vi "Increment Subscribers.vi"(8 "error in (no error)":errorcluster, 11 "CIFChannels in":refnum<class "CIFChannels.lvclass">) -> (0 "error out":errorcluster, 3 "CIFChannels out":refnum<class "CIFChannels.lvclass">)   [LabVIEW 2021, in "CIFChannels.lvclass"]
uses:
  CIFChannels.lvclass
  CIFChannels.lvclass/CIFChannels.ctl
  Typedef/Channel State.ctl
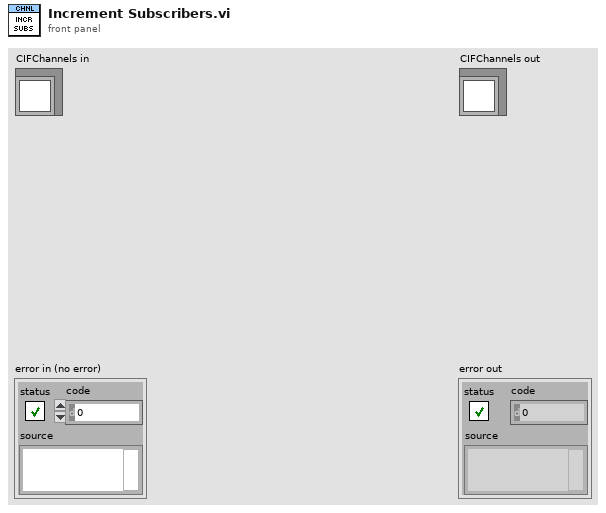
[diagram p1: front panel]
types:
  T1 = typedef "CIFChannels.lvclass/Channel State.ctl" = enum16{"Creating", "Disconnected", "Connecting", "Connected", "Destroyed"}
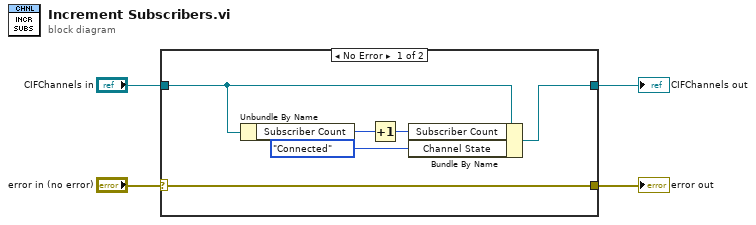
[diagram p0: block diagram]
diagram:
  n1 = case shown="No Error" "error in (no error)" {
    selector: "error in (no error)" -> [w10 w12]
    tunnel: [w10 w12] -> w3
    tunnel: [w5 w11] -> w1
    tunnel: "CIFChannels in" -> [w8 w11]
    frame No Error {
      n2 = Unbundle By Name(w8) -> ("Subscriber Count"=w9:u32)
      n3 = Increment(x=w9) -> (x+1=w7:u32)
      n4 = Bundle By Name(cluster=w8, "Subscriber Count"=w7, "Channel State"=Channel_State."Connected") -> (w5:refnum<class "CIFChannels.lvclass">)
    }
    frame Error {
    }
  }
  "error out" <- w3
  "CIFChannels out" <- w1
